vi "Compute Local Convex Hull.vi"(6 "Included Points":T2[](array[typedef])) -> (1 "Convex Hull":T1[](array[typedef]), 3 "Sorted Array":T1[](array[typedef]))   [LabVIEW 2018, in "Video Cam Processor.lvclass"]
uses:
  Video Cam Processor.lvclass
  Private/Hull Point STYP.ctl
  Shared/Graham Scan/Graham Scan Point.ctl
  3579da19-26b3-4257-af63-783c8511726a.vi
  b6be5d93-7c5a-40d0-8167-307c808ccd24.vi
  d20e1aef-ff1b-49c2-ab5e-746099a590f7.vi
  b6be5d93-7c5a-40d0-8167-307c808ccd24.vi/1833dcaf-1881-4148-8c0a-240b5542455f.vi
  d20e1aef-ff1b-49c2-ab5e-746099a590f7.vi/c0b615b5-2906-4ead-81bf-e15d0bbcd94c.vi
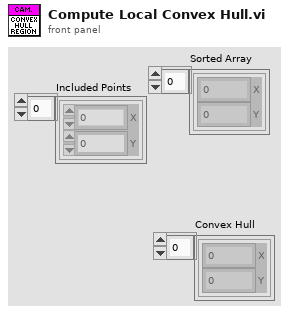
[diagram p1: front panel]
types:
  T1 = typedef "Graham Scan Point.ctl" = cluster{"X":i32, "Y":i32}
  T2 = typedef "Video Cam Processor.lvclass/Hull Point STYP.ctl" = cluster{"X":i32, "Y":i32}
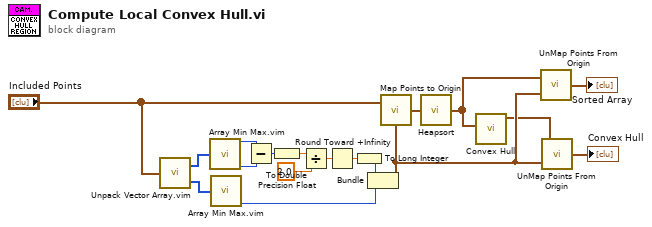
[diagram p0: block diagram]
diagram:
  n1 = call "Unpack Vector Array.vim"("Vector Array"="Included Points") -> ("Y Array"=w9:i32[], "X Array"=w8:i32[])  [unwired: 2 in]
  n2 = call "Array Min Max.vim"("Array"=w8) -> ("Max"=w10:i32, "Min"=w11:i32)  [unwired: 13 in]
  n3 = call "Array Min Max.vim"("Array"=w9) -> ("Min"=w18:i32)  [unwired: 13 in, 1 out]
  n4 = Subtract(x=w10, y=w11) -> (x-y=w12:i32)
  n5 = To Double Precision Float(number=w12) -> (double precision float=w13:dbl)
  n6 = Divide(x=w13, y=2.0) -> (x/y=w15:dbl)
  n7 = Round Toward +Infinity(x=w15) -> (ceil(x): smallest int >= x=w16:dbl)
  n8 = To Long Integer(number=w16) -> (32bit integer=w17:i32)
  n9 = Bundle(w17, "Min"=w18) -> (w6:cluster{i32, "Min":i32})  [unwired: 1 in]
  n10 = call "Map Points to Origin.vi"("New Origin"=w6, "Points"="Included Points") -> ("Mapped Points"=w2:T1[])
  n11 = call "Heapsort.vi"("Array"=w2) -> ("Sorted Array"=w1:T1[])
  n12 = call "Convex Hull.vi"("Sorted Array"=w1) -> ("Convex Hull"=w3:T1[])  [unwired: 5 in, 1 out]
  n13 = call "UnMap Points From Origin.vi"("New Origin"=w6, "Points"=w1) -> ("Mapped Points"=→"Sorted Array":T1[])
  n14 = call "UnMap Points From Origin.vi"("New Origin"=w6, "Points"=w3) -> ("Mapped Points"=→"Convex Hull":T1[])
